vi "to string.vi"(8 "error in":errorcluster, 11 "configuration in":refnum<class "PL_System Configuration.lvclass">) -> (0 "error out":errorcluster, 1 "data":string, 2 "version":string, 3 "configuration out":refnum<class "PL_System Configuration.lvclass">)   [LabVIEW 2013, in "PL_System Configuration.lvclass"]
doc: "Provides an interface for saving a module configuration to a file or other serialized data source. It is recommended that all children of this class store data in two sets--data required for its own initialization, and any data required for parent initialization--and that each implementation uses the <b>Call Parent Method</b> primitive to serialize parent information."
uses:
  PL_System Configuration.lvclass
  <vilib>/NI/Tag Bus Module Framework/root configuration/TBM configuration.lvclass
  PL_System Configuration.lvclass/PL_System Configuration.ctl
  <vilib>/NI/Configuration Framework/serializable configuration/NISE_CEF_serializable configuration.lvclass
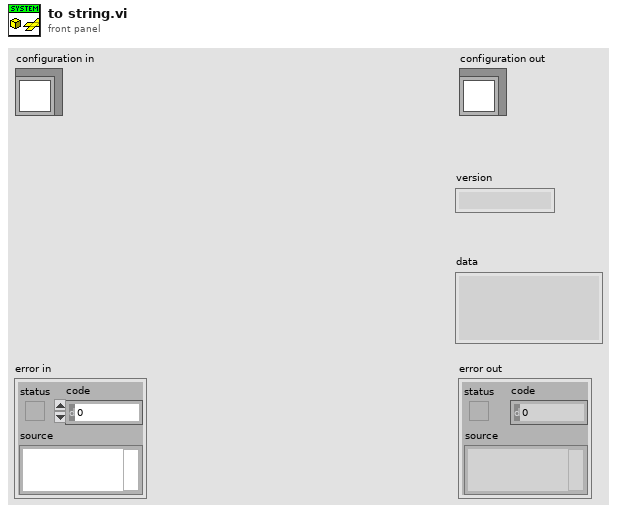
[diagram p1: front panel]
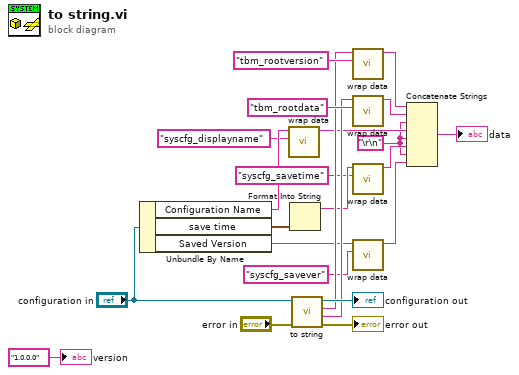
[diagram p0: block diagram]
diagram:
  w4 = "\r\n"
  n1 = Unbundle By Name("configuration in") -> ("Configuration Name"=w11:string, "save time"=w10:timestamp, "Saved Version"=w3:string)
  n2 = call <vilib>:"wrap data.vi"("identifier"="syscfg_displayname" ("additional identifier"), "data to wrap"=w11) -> ("wrapped data"=w6:string)  [unwired: 9 in]
  n3 = Format Into String(w10) -> (resulting string=w9:string)  [unwired: 3 in, 1 out]
  n4 = call-parent "to string.vi"("error in"="error in", "configuration in"="configuration in") -> ("error out"=→"error out":errorcluster, "data"=w12:string, "version"=w13:string, "configuration out"=→"configuration out":refnum<class "PL_System Configuration.lvclass">)  [unwired: 6 in]
  n5 = call <vilib>:"wrap data.vi"("identifier"="tbm_rootversion" ("additional identifier"), "data to wrap"=w13) -> ("wrapped data"=w16:string)  [unwired: 9 in]
  n6 = call <vilib>:"wrap data.vi"("identifier"="tbm_rootdata" ("additional identifier"), "data to wrap"=w12) -> ("wrapped data"=w15:string)  [unwired: 9 in]
  n7 = call <vilib>:"wrap data.vi"("identifier"="syscfg_savetime" ("additional identifier"), "data to wrap"=w9) -> ("wrapped data"=w5:string)  [unwired: 9 in]
  n8 = call <vilib>:"wrap data.vi"("identifier"="syscfg_savever" ("additional identifier"), "data to wrap"=w3) -> ("wrapped data"=w1:string)  [unwired: 9 in]
  n9 = Concatenate Strings(w16, w15, w4, w6, w4, w5, w4, w1) -> (→"data":string)
  "version" <- "1.0.0.0" ("version")
